vi "insertEntlogFromEntlogTmp.vi"() -> ()   [LabVIEW 2012]
uses:
  <vilib>/addons/database/Connection.llb/DB Tools Open Connec (Path).vi
  <vilib>/addons/database/Connection.llb/Conn Execute.vi
  <vilib>/addons/database/Recordset.llb/Rec Fetch Recordset Data (R).vi
  <vilib>/addons/database/Recordset.llb/Rec Destroy - Connection.vi
  <vilib>/addons/database/_DB Variant To Data/Database Variant To Data.xnode
  <vilib>/addons/database/NI_Database_API.lvlib
panel:
  out "error out 3":errorcluster
  out "recordset data":variant[][](array[variant])
  out "concatenated string":string
  out "concatenated string 2":string
  out "time stamp":timestamp
  out "time stamp 2":timestamp
  out "error out":errorcluster
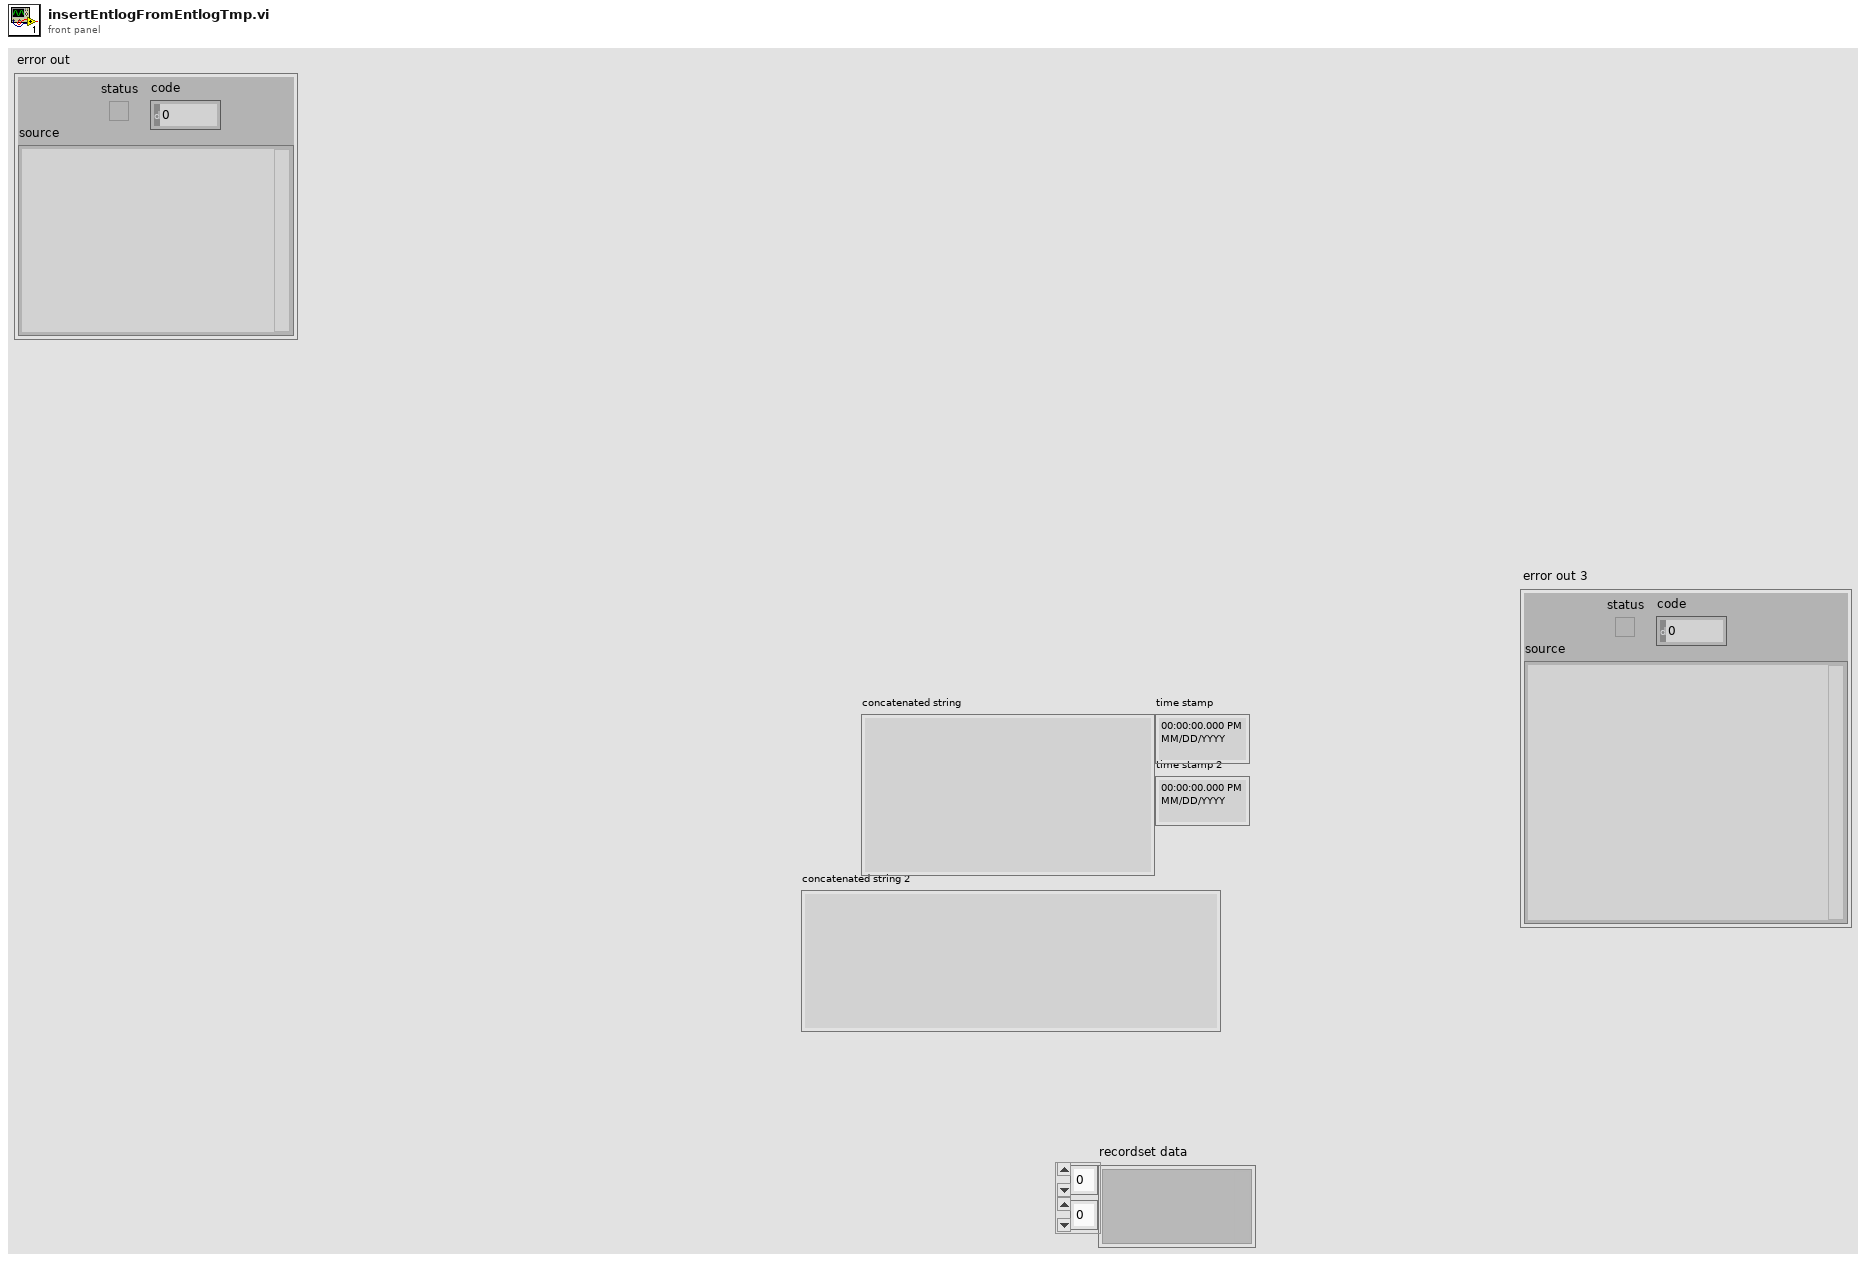
[diagram p1: front panel]
types:
  T1 = typedef "NI_Database_API.lvlib/Conn ObjectReference.ctl" = refnum<k1>
  T2 = typedef "NI_Database_API.lvlib/Rec ObjectReference.ctl" = refnum<k1>
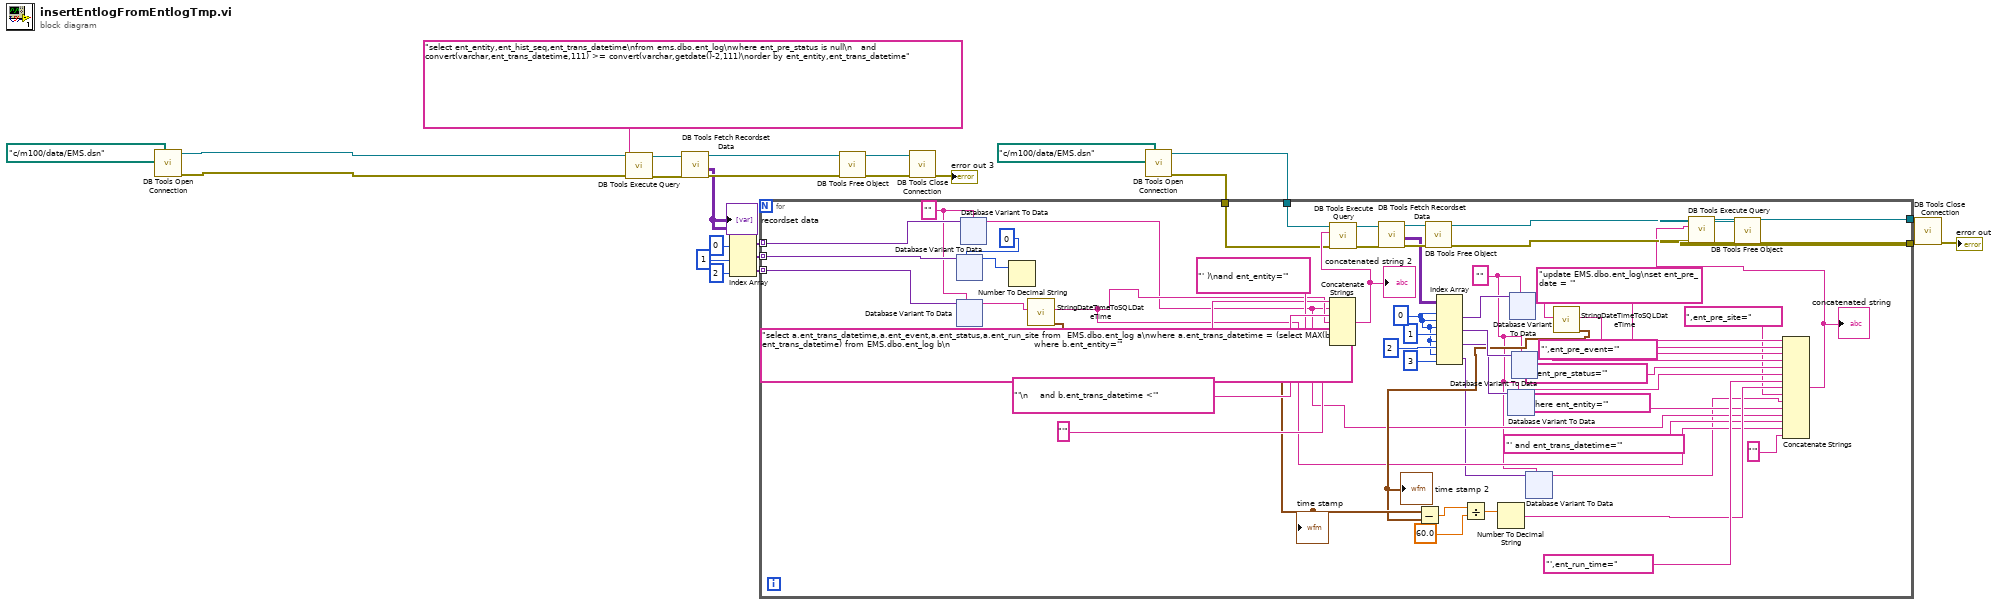
[diagram p0: block diagram]
diagram:
  n1 = call-poly <vilib>:"DB Tools Open Connection.vi"("connection information"=path "c:/m100/data/EMS.dsn") -> ("error out"=w1:errorcluster, "connection reference"=w2:T1)  [unwired: 7 in]
  n2 = call-poly <vilib>:"DB Tools Execute Query.vi"("error in (no error)"=w1, "SQL query"="select ent_entity,ent_hist_seq,ent_trans_datetime\nfrom ems.dbo.ent_log\nwhere ent_pre_status is null\n   and convert(varchar,ent_trans_datetime,111) >= convert(varchar,getdate()-2,111)\norder by ent_entity,ent_trans_datetime", "connection reference"=w2) -> ("error out"=w22:errorcluster, "recordset reference"=w24:T2)  [unwired: 5 in]
  n3 = call-poly <vilib>:"DB Tools Fetch Recordset Data.vi"("error in (no error)"=w22, "recordset reference"=w24) -> ("error out"=w21:errorcluster, "recordset data"=w18:variant[][], "recordset reference out"=w23:T2)  [unwired: 3 in]
  "recordset data" <- w18
  n4 = Index Array(array=w18, index (col) #1=0 ("disabled index (col)"), index (col) #2=1 ("index (col)"), index (col) #3=2 ("index (col)")) -> (element #1=w17:variant[], element #2=w16:variant[], element #3=w15:variant[])  [unwired: 3 in]
  n5 = call-poly <vilib>:"DB Tools Free Object.vi"("error in (no error)"=w21, "recordset reference"=w23) -> ("error out"=w10:errorcluster, "connection reference"=w11:T1)  [unwired: 8 in]
  n6 = call <vilib>:"DB Tools Close Connection.vi"("error in (no error)"=w10, "connection reference"=w11) -> ("error out"=→"error out 3":errorcluster)  [unwired: 5 in]
  n7 = call-poly <vilib>:"DB Tools Open Connection.vi"("connection information"=path "c:/m100/data/EMS.dsn") -> ("error out"=w8:errorcluster, "connection reference"=w9:T1)  [unwired: 7 in]
  n8 = for {
    tunnel: w17 -> [w80] mode=indexing
    tunnel: w16 -> [w79] mode=indexing
    tunnel: w15 -> [w78] mode=indexing
    tunnel: [w68] -> w14
    tunnel: w9 -> [w73]
    tunnel: w8 -> [w71]
    tunnel: [w67] -> w3
    w26 = ""
    w28 = 0 ("disabled index (col)")
    w38 = ""
    n9 = xnode "Database Variant To Data"("database variant"=w79, "type"=0) -> ("data"=w36:i32)  [unwired: 1 in, 1 out]
    n10 = xnode "Database Variant To Data"("database variant"=w78, "type"=w38) -> ("data"=w76:string)  [unwired: 1 in, 1 out]
    n11 = xnode "Database Variant To Data"("database variant"=w80, "type"=w38) -> ("data"=w31:string)  [unwired: 1 in, 1 out]
    n12 = Number To Decimal String(number=w36) -> ()  [unwired: 1 in, 1 out]
    n13 = call "StringDateTimeToSQLDateTime.vi"("String"=w76) -> ("time stamp"=w45:timestamp, "date/time string"=w33:string)  [unwired: 9 in]
    "time stamp" <- w45
    n14 = Concatenate Strings("select a.ent_trans_datetime,a.ent_event,a.ent_status,a.ent_run_site from  EMS.dbo.ent_log a\nwhere a.ent_trans_datetime = (select MAX(b.ent_trans_datetime) from EMS.dbo.ent_log b\n                            where b.ent_entity='" ("string"), w31, "'\n    and b.ent_trans_datetime <'" ("string"), w33, "' )\nand ent_entity='" ("string"), w31, "'") -> (w72:string)
    "concatenated string 2" <- w72
    n15 = call-poly <vilib>:"DB Tools Execute Query.vi"("error in (no error)"=w71, "SQL query"=w72, "connection reference"=w73) -> ("error out"=w63:errorcluster, "recordset reference"=w64:T2)  [unwired: 5 in]
    n16 = call-poly <vilib>:"DB Tools Fetch Recordset Data.vi"("error in (no error)"=w63, "recordset reference"=w64) -> ("error out"=w65:errorcluster, "recordset data"=w60:variant[][], "recordset reference out"=w66:T2)  [unwired: 3 in]
    n17 = call-poly <vilib>:"DB Tools Free Object.vi"("error in (no error)"=w65, "recordset reference"=w66) -> ("error out"=w61:errorcluster, "connection reference"=w62:T1)  [unwired: 8 in]
    n18 = Index Array(array=w60, index (row) #1=w28, index (col) #1=w28, index (row) #2=w28, index (col) #2=1 ("index (col)"), index (row) #3=w28, index (col) #3=2 ("index (col)"), index (row) #4=w28, index (col) #4=3 ("index (col)")) -> (element #1=w56:variant, element #2=w52:variant, element #3=w49:variant, element #4=w27:variant)
    n19 = xnode "Database Variant To Data"("database variant"=w49, "type"=w26) -> ("data"=w48:string)  [unwired: 1 in, 1 out]
    n20 = xnode "Database Variant To Data"("database variant"=w56, "type"=w26) -> ("data"=w55:string)  [unwired: 1 in, 1 out]
    n21 = xnode "Database Variant To Data"("database variant"=w52, "type"=w26) -> ("data"=w51:string)  [unwired: 1 in, 1 out]
    n22 = xnode "Database Variant To Data"("database variant"=w27, "type"=w26) -> ("data"=w25:string)  [unwired: 1 in, 1 out]
    n23 = call "StringDateTimeToSQLDateTime.vi"("String"=w55) -> ("time stamp"=w44:timestamp, "date/time string"=w54:string)  [unwired: 9 in]
    "time stamp 2" <- w44
    n24 = Subtract(x=w45, y=w44) -> (x-y=w43:dbl)
    n25 = Divide(x=w43, y=60.0) -> (x/y=w40:dbl)
    n26 = Number To Decimal String(number=w40) -> (decimal integer string=w39:string)  [unwired: 1 in]
    n27 = Concatenate Strings("update EMS.dbo.ent_log\nset ent_pre_date = '" ("string"), w54, "',ent_pre_event='" ("string"), w51, "',ent_pre_status='" ("string"), w48, "',ent_run_time=", w39, ",ent_pre_site=" ("string"), w25, " where ent_entity='" ("string"), w31, "' and ent_trans_datetime='" ("string"), w33, "'" ("string")) -> (w47:string)
    "concatenated string" <- w47
    n28 = call-poly <vilib>:"DB Tools Execute Query.vi"("error in (no error)"=w61, "SQL query"=w47, "connection reference"=w62) -> ("error out"=w69:errorcluster, "recordset reference"=w70:T2)  [unwired: 5 in]
    n29 = call-poly <vilib>:"DB Tools Free Object.vi"("error in (no error)"=w69, "recordset reference"=w70) -> ("error out"=w67:errorcluster, "connection reference"=w68:T1)  [unwired: 8 in]
  }
  n30 = call <vilib>:"DB Tools Close Connection.vi"("error in (no error)"=w3, "connection reference"=w14) -> ("error out"=→"error out":errorcluster)  [unwired: 5 in]
